vi "ShooterWheelLogicV3.vi"(0 "Setpoint":dbl, 5 "Process Varaible":dbl, 7 "Feedfoward Voltage":dbl, 9 "SwitchZones":T1, 11 "PID gains":T2, 12 "Error Margin":dbl, 13 "Reset":bool) -> (4 "At Speed":bool, 6 "Motor Output":dbl, 8 "Voltage Output":dbl, 10 "Error":dbl, 15 "Wheel Died":bool)   [LabVIEW 2012]
uses:
  Max'sToolKit/ConvertVoltageToPercentVbs.vi
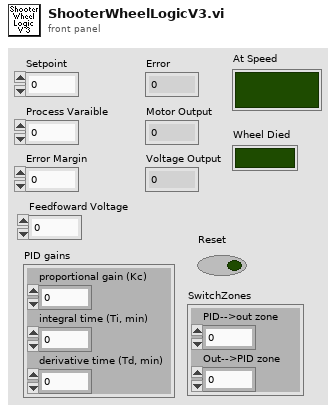
[diagram p1: front panel]
types:
  T1 = cluster{"PID-->out zone":dbl, "Out-->PID zone":dbl}
  T2 = cluster{"proportional gain (Kc)":dbl, "integral time (Ti, min)":dbl, "derivative time (Td, min)":dbl}
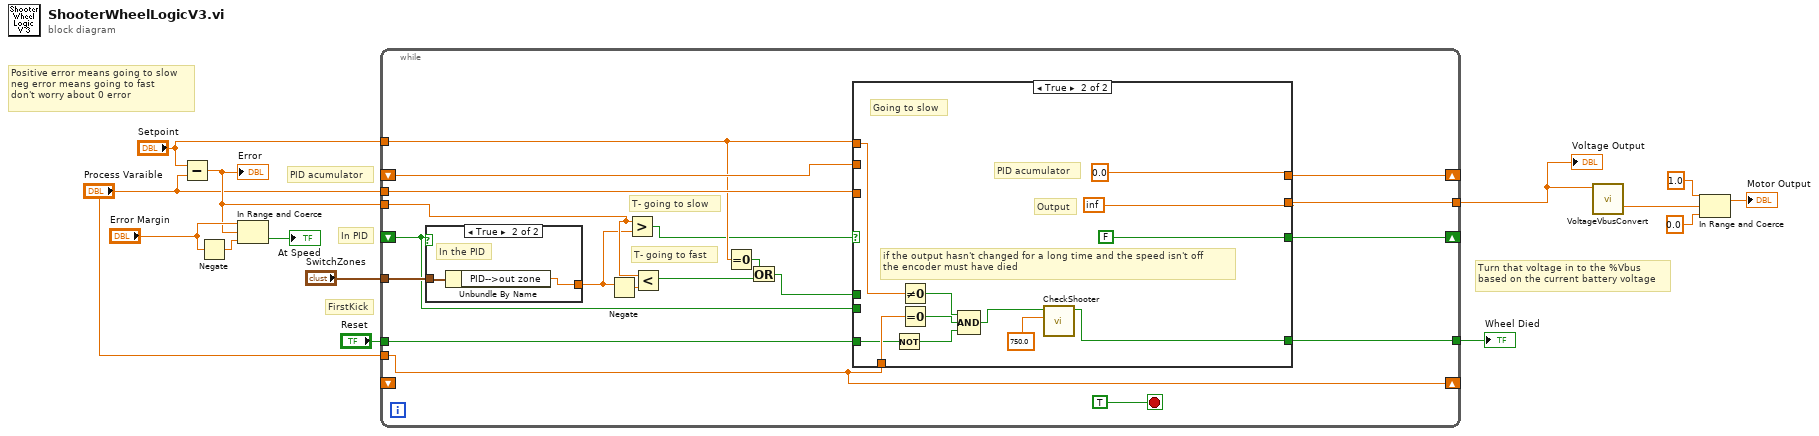
[diagram p0: block diagram]
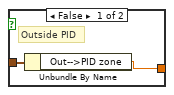
[diagram p2: hidden frame]
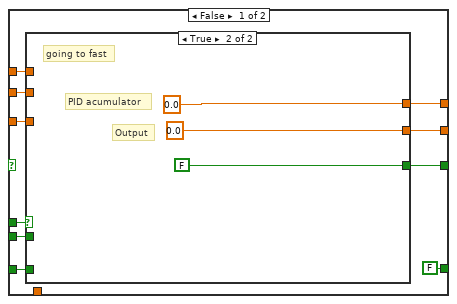
[diagram p3: hidden frame]
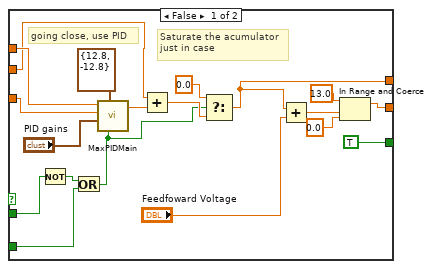
[diagram p4: hidden frame]
diagram:
  # "Turn that voltage in to the %Vbus\nbased on the current battery voltage"
  # "In PID"
  # "PID acumulator"
  # "FirstKick"
  # "Positive error means going to slow\nneg error means going to fast\ndon't worry about 0 error"
  n1 = Subtract(x="Setpoint", y="Process Varaible") -> (x-y=w4:dbl)
  "Error" <- w4
  n2 = Negate(x="Error Margin") -> (-x=w11:dbl)
  n3 = In Range and Coerce(upper limit="Error Margin", x=w4, lower limit=w11) -> (In Range?=→"At Speed":bool)  [unwired: 1 out]
  n4 = while {
    tunnel: "Setpoint" -> [w23]
    tunnel: "Process Varaible" -> [w33]
    tunnel: "Reset" -> [w32]
    shift-right: [w29] -> _
    shift-left: _ -> [w30]
    tunnel: [w28] -> w6
    shift-right: [w27] -> _
    shift-left: _ -> [w15]
    tunnel: w4 -> [w20]
    tunnel: "Process Varaible" -> [w18]
    shift-right: [w18] -> _
    shift-left: _ -> [_]
    tunnel: "SwitchZones" -> [w17]
    tunnel: [w16] -> w1
    stop <- TRUE stop-if-true
    # "T- going to fast"
    # "T- going to slow"
    n5 = case shown="True" w15 {
      tunnel: [w34 w37] -> w19
      tunnel: w17 -> [w35 w36]
      frame False {
        # "Outside PID"
        n6 = Unbundle By Name(w35) -> ("Out-->PID zone"=w34:dbl)
      }
      frame True {
        # "In the PID"
        n7 = Unbundle By Name(w36) -> ("PID-->out zone"=w37:dbl)
      }
    }
    n8 = Negate(x=w19) -> (-x=w24:dbl)
    n9 = Greater?(x=w20, y=w19) -> (0:w21:bool)
    n10 = Less?(x=w20, y=w24) -> (x < y?=w25:bool)
    n11 = Equal To 0?(x=w23) -> (x = 0?=w26:bool)
    n12 = Or(x=w26, y=w25) -> (x .or. y?=w22:bool)
    n13 = case shown="True" w21 {
      tunnel: w22 -> [w47 _]
      tunnel: w23 -> [w46 w76]
      tunnel: w33 -> [w45 _]
      tunnel: w32 -> [w44 w74]
      tunnel: w30 -> [w43 _]
      tunnel: [w42 0.0 ("lower limit")] -> w29
      tunnel: [w41 inf] -> w28
      tunnel: [w40 FALSE] -> w27
      tunnel: w18 -> [_ w75]
      tunnel: [FALSE ("Good to shoot") w77] -> w16
      tunnel: w15 -> [w38 _]
      frame False {
        n14 = case shown="True" w47 {
          tunnel: w46 -> [w64 _]
          tunnel: w45 -> [w63 _]
          tunnel: w44 -> [w50 _]
          tunnel: w43 -> [w58 _]
          tunnel: [w54 0.0 ("lower limit")] -> w42
          tunnel: [w52 0.0 ("lower limit")] -> w41
          tunnel: [TRUE FALSE] -> w40
          tunnel: w38 -> [w48 _]
          frame False {
            # "Saturate the acumulator\njust in case"
            # "going close, use PID"
            n15 = Not(x=w48) -> (.not. x?=w49:bool)
            n16 = Or(x=w49, y=w50) -> (x .or. y?=w51:bool)
            n17 = call "MaxPIDMain.vi"("Reset"=w51, "Output Range"=cluster{"output high":dbl, "output low":dbl} {"output high"=12.8, "output low"=-12.8} ("output range"), "PID gains"="PID gains", "process variable"=w63, "setpoint"=w64) -> ("Output"=w61:dbl)  [unwired: 5 in, 1 out]
            n18 = Add(x=w58, y=w61) -> (x+y=w56:dbl)
            n19 = Select(t=0.0 ("lower limit"), s=w51, f=w56) -> (s? t:f=w54:dbl)
            n20 = Add(x=w54, y="Feedfoward Voltage") -> (x+y=w55:dbl)
            n21 = In Range and Coerce(upper limit=13.0, x=w55, lower limit=0.0) -> (coerced(x)=w52:dbl)  [unwired: 1 out]
          }
          frame True {
            # "Output"
            # "PID acumulator"
            # "going to fast"
          }
        }
      }
      frame True {
        # "if the output hasn't changed for a long time and the speed isn't off\nthe encoder must have died"
        # "Output"
        # "PID acumulator"
        # "Going to slow"
        n22 = Not(x=w74) -> (.not. x?=w73:bool)
        n23 = Not Equal To 0?(x=w76) -> (x != 0?=w71:bool)
        n24 = Equal To 0?(x=w75) -> (x = 0?=w72:bool)
        n25 = Compound Arithmetic op=AND(w71, w72, w73) -> (w70:bool)
        n26 = call "CheckShooter.vi"("Time for happy (ms)"=750.0, "Shooter Good?"=w70) -> ("Good to shoot"=w77:bool)  [unwired: 9 in]
      }
    }
  }
  "Voltage Output" <- w6
  "Wheel Died" <- w1
  n27 = call-poly "VoltageVbusConvert.vi"("Voltage"=w6) -> ("Vbus"=w8:dbl)  [unwired: 10 in]
  n28 = In Range and Coerce(upper limit=1.0, x=w8, lower limit=0.0) -> (coerced(x)=→"Motor Output":dbl)  [unwired: 1 out]
